vi "Actor Core.vi"(8 "error in":errorcluster, 11 "Measure Object in":refnum<class "Measure App.lvclass">) -> (0 "error out":errorcluster, 3 "Actor out":refnum<class "Actor.lvclass">)   [LabVIEW 2018, in "Measure App.lvclass"]
doc: "(<B>Filename</B>: Actor Framework.lvlib:Actor.lvclass:Actor Core.vi)\n\nReceives messages to the actor, reacts to them, and initiates any error handling that may shut the actor down.\n\nDescendant classes may override this VI to append parallel tasks for the actor to complete while it handles messages. Overrides use the Call Parent Method node."
uses:
  Measure App.lvclass
  C:/github/LabActor/Template Module/Template Module.lvclass
  C:/Program Files/National Instruments/LabVIEW 2018/vi.lib/ActorFramework/Actor/Actor.lvclass
  <vilib>/ActorFramework/Actor/Actor.lvclass
  Measure App.lvclass/Measure App.ctl
  Template Module/Template Module.lvclass/Template Module.ctl
  <vilib>/ActorFramework/Actor/Actor.lvclass/Actor.ctl
  <vilib>/ActorFramework/Message Enqueuer/Message Enqueuer.lvclass/Message Enqueuer.ctl
  <vilib>/Utility/sysdir.llb/System Directory Type.ctl
  Template Module Messages/Save Configuration Msg/Save Configuration Msg.lvclass/Save Configuration Msg.ctl
  Plots/Plot types.ctl
  Controllers/Application Controller Messages/Open Waveform File Plot Msg/Open Waveform File Plot Msg.lvclass/Open Waveform File Plot Msg.ctl
  LabActor Messages/Stop Measurements Command Msg/Stop Measurements Command Msg.lvclass/Stop Measurements Command Msg.ctl
  Template Module/Read stop event.vi
  <vilib>/ActorFramework/Message Enqueuer/Init from Existing Queue.vi
  <vilib>/ActorFramework/Message Enqueuer/Enqueue.vi
  <vilib>/ActorFramework/Stop Msg/Stop Msg.lvclass
  C:/Program Files/National Instruments/LabVIEW 2018/vi.lib/ActorFramework/Message/Message.lvclass
  Template Module Messages/Save Configuration Msg/Save Configuration Msg.lvclass
  Controllers/Application Controller Messages/Open Waveform File Plot Msg/Open Waveform File Plot Msg.lvclass
  LabActor Messages/Stop Measurements Command Msg/Stop Measurements Command Msg.lvclass
  <vilib>/ActorFramework/Message Priority Queue/Priority Enqueue.vi
  Controllers/Application Controller/Application Controller.lvclass
  <vilib>/ActorFramework/Message Enqueuer/Message Enqueuer.lvclass
  Template Module Messages/Restore Configuration Msg/Restore Configuration Msg.lvclass
panel:
  out "Monitor file":path caption="Current\nFile"
  in  "Stop monitor":bool
  in  "View Waveform":bool
  in  "Full XY Plot":bool
  in  "View XY Plot":bool
  in  "Read cfg":bool
  in  "Write cfg":bool
  in  "Exit":bool
  out "Pulse file":path caption="Last\nFile"
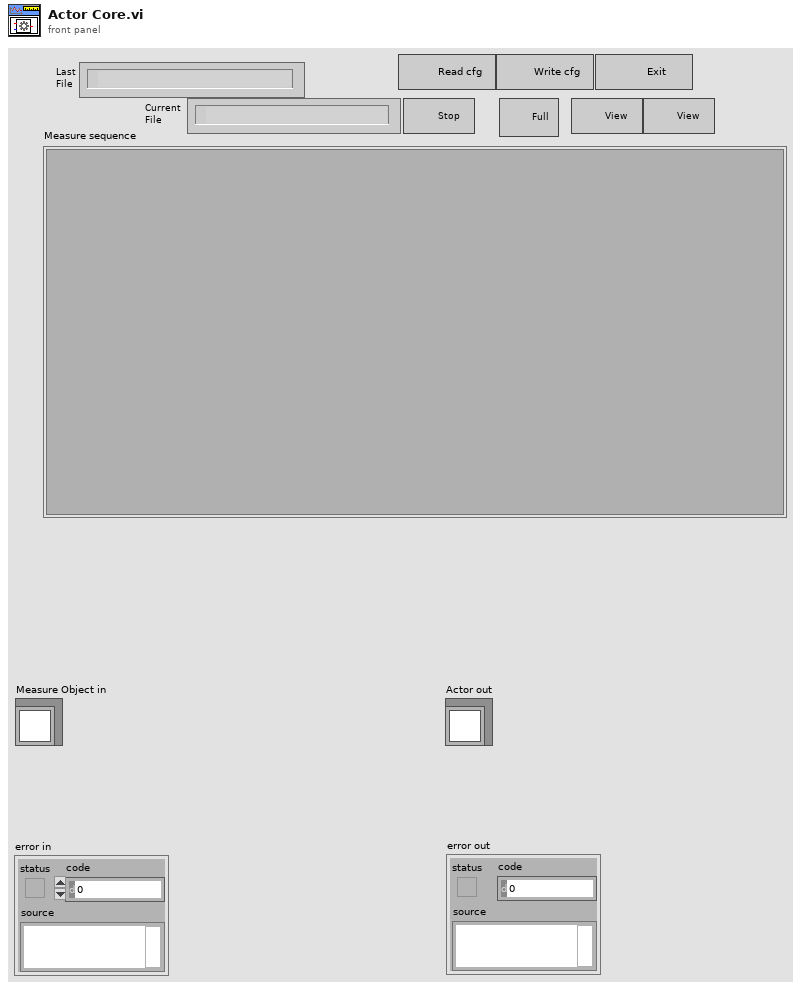
[diagram p1: front panel]
types:
  T1 = typedef "Plot types.ctl" = enum16{"Waveform Plot", "XY Plot", "Full XY"}
  T2 = typedef "System Directory Type.ctl" = i32
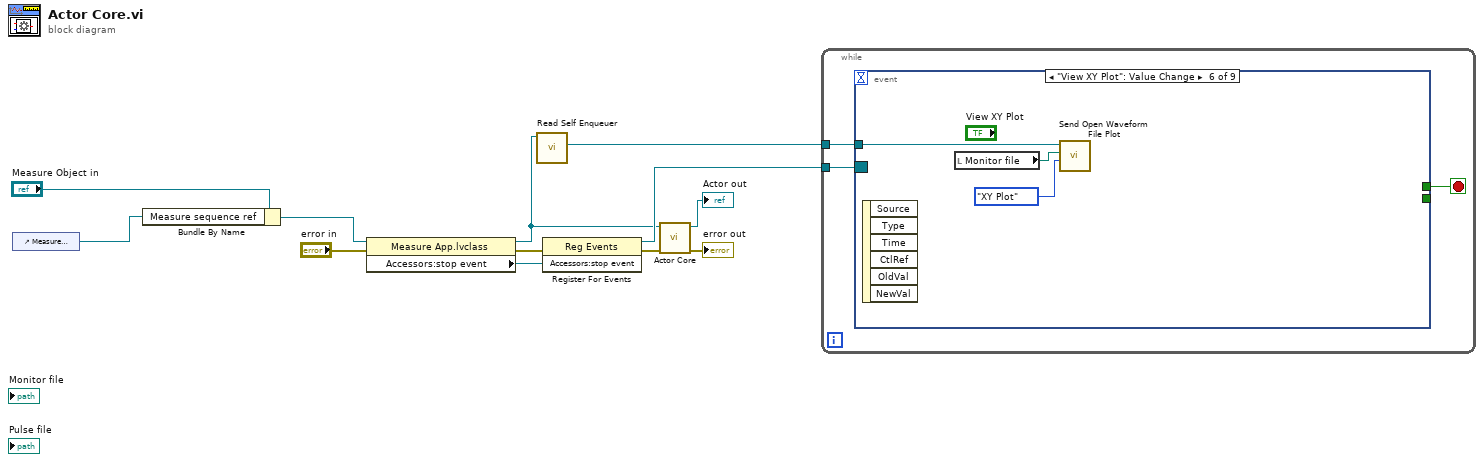
[diagram p0: block diagram]
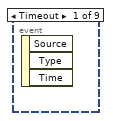
[diagram p2: hidden frame]
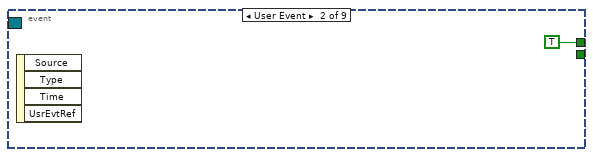
[diagram p3: hidden frame]
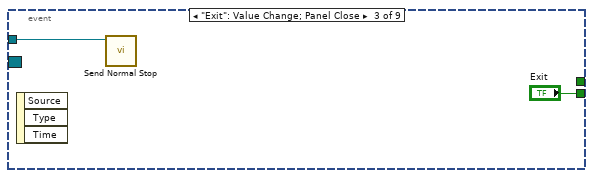
[diagram p4: hidden frame]
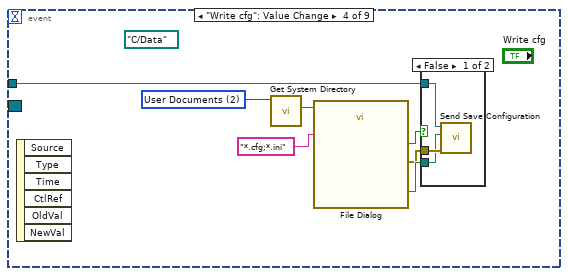
[diagram p5: hidden frame]
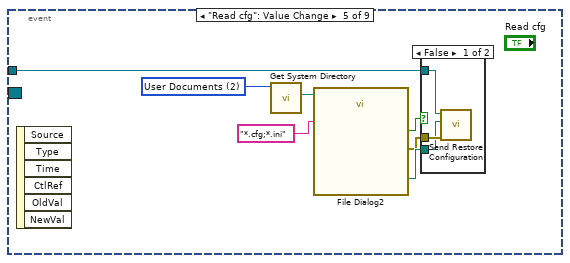
[diagram p7: hidden frame]
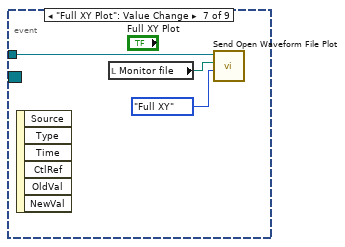
[diagram p9: hidden frame]
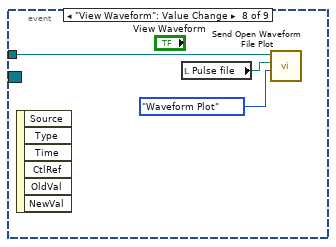
[diagram p10: hidden frame]
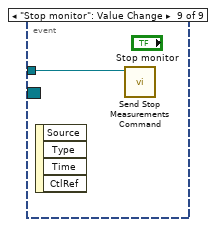
[diagram p11: hidden frame]
diagram:
  n1 = control-ref of="Measure sequence"() -> (w9:refnum<vi>)
  n2 = Bundle By Name(cluster="Measure Object in", "Measure sequence ref"=w9) -> (w5:refnum<class "Measure App.lvclass">)
  n3 = property class="Measure App.lvclass"(reference=w5, error in="error in") -> (reference out=w1:refnum<class "Measure App.lvclass">, error out=w7:errorcluster, "Accessors:stop event"=w2:refnum<user-event>)
  n4 = call <vilib>:"Read Self Enqueuer.vi"("Actor"=w1) -> ("Self Enqueuer"=w6:refnum<class "Message Enqueuer.lvclass">)  [unwired: 10 in]
  n5 = register-events(error in=w7, w2) -> (reference out=w8:refnum<event-registration>, error out=w3:errorcluster)  [unwired: 1 in]
  n6 = call-parent "Actor Core.vi"("error in"=w3, "Measure Object in"=w1) -> ("error out"=→"error out":errorcluster, "Actor out"=→"Actor out":refnum<class "Actor.lvclass">)  [unwired: 8 in]
  n7 = while {
    tunnel: w8 -> [w15]
    tunnel: w6 -> [w13]
    stop <- w14 stop-if-true
    n8 = event shown="[5] \"View XY Plot\": Value Change" {
      selector: w15 -> [_ _ _ _ _ _ _ _ _]
      dyn-events: _ -> [_ _ _ _ _ _ _ _ _]
      timeout: _ -> [_ _ _ _ _ _ _ _ _]
      tunnel: [_ TRUE _ _ _ _ _ _ _] -> w14
      tunnel: w13 -> [_ _ w17 w22 w30 w41 w44 w46 w48]
      tunnel: [_ _ "Exit" _ _ _ _ _ _] -> _
      event Timeout {
        n9 = event-data() -> ()  [unwired: 1 in, 3 out]
      }
      event User Event {
        n10 = event-data() -> ()  [unwired: 1 in, 4 out]
      }
      event "Exit": Value Change; Panel Close {
        n11 = event-data() -> ()  [unwired: 1 in, 3 out]
        n12 = call <vilib>:"Send Normal Stop.vi"("Message Enqueuer"=w17) -> ()  [unwired: 10 in, 1 out]
      }
      event "Write cfg": Value Change {
        w20 = T2 2 items=["User Home"=0, "User Desktop"=1, "User Documents"=2, "User Application Data"=3, "User Preferences"=4, "User Temporary"=5, "Public Documents"=6, "Public Application Data"=7, "Public Preferences"=8, "Public Cache"=13, "System Core Libraries"=9, "System Installed Libraries"=10, "Application Files"=11, "Boot Volume Root"=12] ("system directory type")
        (unwired) path "C:/Data" ("start path")
        n13 = event-data() -> ()  [unwired: 1 in, 6 out]
        n14 = call <vilib>:"Get System Directory.vi"("system directory type"=w20) -> ("system directory"=w19:path)  [unwired: 10 in]
        n15 = call "File Dialog"("start path"=w19, "pattern (all files)"="*.cfg;*.ini") -> ("selected path"=w24:path, "cancelled"=w25:bool, "error out"=w21:errorcluster)  [unwired: 10 in, 1 out]
        n16 = case shown="False" w25 {
          tunnel: w24 -> [w26 _]
          tunnel: w22 -> [w28 _]
          tunnel: w21 -> [w27 _]
          frame False {
            n17 = call "Send Save Configuration.vi"("error in (no error)"=w27, "File path"=w26, "Message Enqueuer"=w28) -> ()  [unwired: 7 in, 2 out]
          }
          frame True {
          }
        }
      }
      event "Read cfg": Value Change {
        w32 = T2 2 items=["User Home"=0, "User Desktop"=1, "User Documents"=2, "User Application Data"=3, "User Preferences"=4, "User Temporary"=5, "Public Documents"=6, "Public Application Data"=7, "Public Preferences"=8, "Public Cache"=13, "System Core Libraries"=9, "System Installed Libraries"=10, "Application Files"=11, "Boot Volume Root"=12] ("system directory type")
        n18 = event-data() -> ()  [unwired: 1 in, 6 out]
        n19 = call <vilib>:"Get System Directory.vi"("system directory type"=w32) -> ("system directory"=w31:path)  [unwired: 10 in]
        n20 = call "File Dialog2"("start path"=w31, "pattern (all files)"="*.cfg;*.ini") -> ("selected path"=w35:path, "cancelled"=w29:bool, "error out"=w33:errorcluster)  [unwired: 10 in, 1 out]
        n21 = case shown="False" w29 {
          tunnel: w35 -> [w36 _]
          tunnel: w30 -> [w38 _]
          tunnel: w33 -> [w37 _]
          frame False {
            n22 = call "Send Restore Configuration.vi"("error in (no error)"=w37, "File path"=w36, "Message Enqueuer"=w38) -> ()  [unwired: 7 in, 2 out]
          }
          frame True {
          }
        }
      }
      event "View XY Plot": Value Change {
        n23 = event-data() -> ()  [unwired: 1 in, 6 out]
        n24 = local read "Monitor file"() -> (w40:path)
        n25 = call "Send Open Waveform File Plot.vi"("Plot type"=Plot_types."XY Plot", "File Path Control"=w40, "Message Enqueuer"=w41) -> ()  [unwired: 7 in, 2 out]
      }
      event "Full XY Plot": Value Change {
        n26 = event-data() -> ()  [unwired: 1 in, 6 out]
        n27 = local read "Monitor file"() -> (w43:path)
        n28 = call "Send Open Waveform File Plot.vi"("Plot type"=Plot_types."Full XY", "File Path Control"=w43, "Message Enqueuer"=w44) -> ()  [unwired: 7 in, 2 out]
      }
      event "View Waveform": Value Change {
        n29 = event-data() -> ()  [unwired: 1 in, 6 out]
        n30 = local read "Pulse file"() -> (w45:path)
        n31 = call "Send Open Waveform File Plot.vi"("Plot type"=Plot_types."Waveform Plot", "File Path Control"=w45, "Message Enqueuer"=w46) -> ()  [unwired: 7 in, 2 out]
      }
      event "Stop monitor": Value Change {
        n32 = event-data() -> ()  [unwired: 1 in, 4 out]
        n33 = call "Send Stop Measurements Command.vi"("Message Enqueuer"=w48) -> ()  [unwired: 9 in, 2 out]
      }
    }
  }
